vi "Close piezo.vi"(8 "Piezo error in":errorcluster, 11 "Piezo handle":i32) -> (0 "error out":errorcluster)   [LabVIEW 2017]
uses:
  <instrlib>/Thorlabs_MDT69xB/Thorlabs_MDT69xB.lvlib
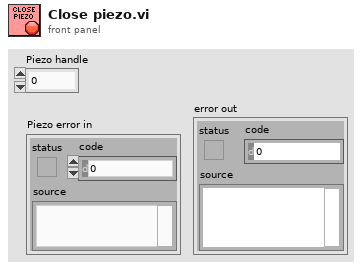
[diagram p1: front panel]
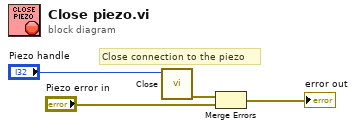
[diagram p0: block diagram]
diagram:
  # "Close connection to the piezo"
  n1 = call <instrlib>:"Close.vi"("hDevice"="Piezo handle") -> ("error out"=w2:errorcluster)  [unwired: 10 in]
  n2 = Merge Errors(w2, "Piezo error in") -> (→"error out":errorcluster)
